vi "S2DS_Update X Y Channel from scan parameters.vi"(7 "Scan parameters in":T1 {"Y data taking" items=["in both direction", "in up direction only", "in down direction only"]; "X data taking" items=["in both direction", "in up direction only", "in down direction only"]}, 9 "WC info in":T2, 10 "Write channel parameters (in)":dbl[][](array[numeric])) -> (1 "WC info out":T2)   [LabVIEW 2025]
uses:
  TYPE DEFS/S2DS_WC info.ctl
  TYPE DEFS/S2DS_Single WC info.ctl
  TYPE DEFS/S2DS_Sweep Info.ctl
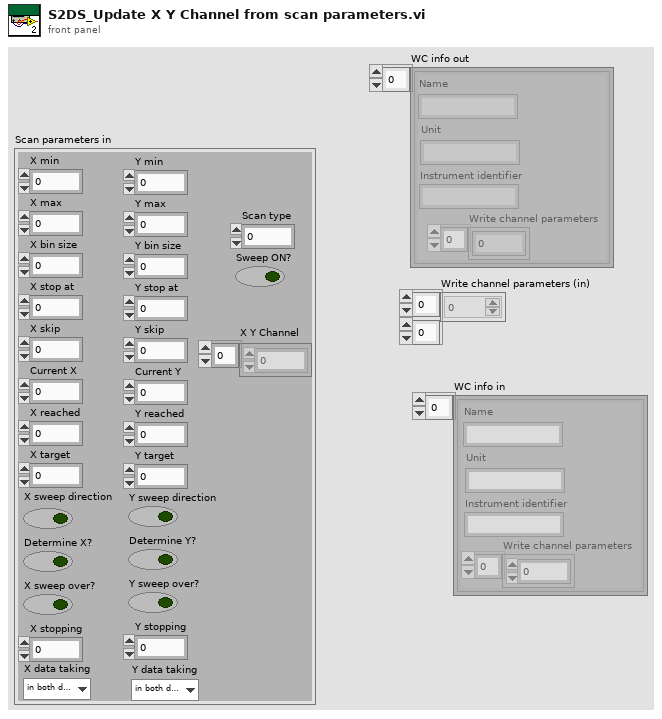
[diagram p1: front panel]
types:
  T1 = typedef "S2DS_Sweep Info.ctl" = cluster{"X min":ext, "X max":dbl, "Y min":dbl, "Y max":dbl, "X bin size":dbl, "Y bin size":dbl, "X stop at":dbl, "Y stop at":dbl, "X skip":u64, "Y skip":u64, "Current X":dbl, "Current Y":dbl, "X reached":i32, "Y reached":i32, "X target":dbl, "Y target":dbl, "Sweep ON?":bool, "X sweep direction":bool, "Y sweep direction":bool, "Determine X?":bool, "Determine Y?":bool, "X sweep over?":bool, "Y sweep over?":bool, "Scan type":i32, "X stopping":i32, "Y stopping":i32, "X Y Channel":u16[], "X data taking":u16, "Y data taking":u16}
  T2 = typedef "S2DS_WC info.ctl" = T3[]
  T3 = typedef "S2DS_Single WC info.ctl" = cluster{"Instrument identifier":string, "Write channel parameters":dbl[], "Name":string, "Unit":string}
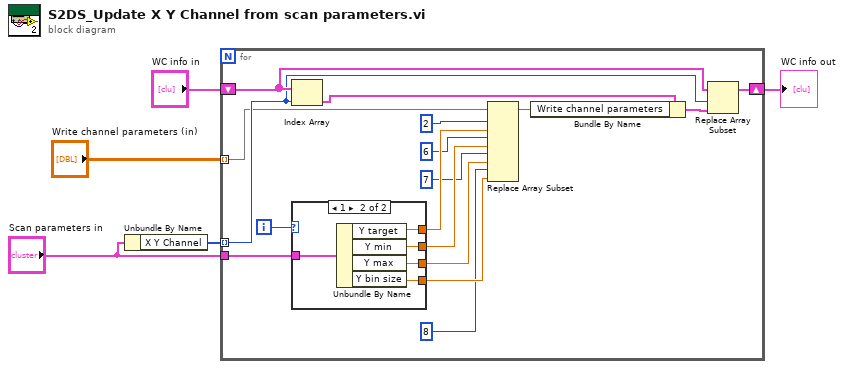
[diagram p0: block diagram]
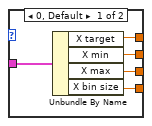
[diagram p2: hidden frame]
diagram:
  n1 = Unbundle By Name("Scan parameters in") -> ("X Y Channel"=w1:u16[])
  n2 = for {
    tunnel: "Write channel parameters (in)" -> [w17] mode=indexing
    shift-right: [w18] -> w4
    shift-left: "WC info in" -> [w21]
    tunnel: w1 -> [w19] mode=indexing
    tunnel: "Scan parameters in" -> [w14]
    i -> [w15]
    n3 = Index Array(array=w21, index=w19) -> (element=w22:T3)
    n4 = case shown="1" w15 {
      tunnel: w14 -> [w27 w32]
      tunnel: [w26 w31] -> w13
      tunnel: [w25 w30] -> w10
      tunnel: [w24 w29] -> w9
      tunnel: [w23 w28] -> w8
      frame 0, Default {
        n5 = Unbundle By Name(w27) -> ("X target"=w26:dbl, "X min"=w25:ext, "X max"=w24:dbl, "X bin size"=w23:dbl)
      }
      frame 1 {
        n6 = Unbundle By Name(w32) -> ("Y target"=w31:dbl, "Y min"=w30:dbl, "Y max"=w29:dbl, "Y bin size"=w28:dbl)
      }
    }
    n7 = Replace Array Subset(array=w17, new element #1=w13, index #1=2 ("index"), new element #2=w10, index #2=6 ("index"), new element #3=w9, index #3=7 ("index"), new element #4=w8, index #4=8 ("index")) -> (w12:dbl[])
    n8 = Bundle By Name(cluster=w22, "Write channel parameters"=w12) -> (w20:T3)
    n9 = Replace Array Subset(array=w21, new element=w20, index=w19) -> (w18:T2)
  }
  "WC info out" <- w4
